vi "MeasureLeakage.vi"(5 "Junction Name":string, 6 "UiDefinition":T1, 7 ".NET Refnum":refnum<k24>, 8 "new file path (Not A Path if cancelled)":path, 9 "appended path":path, 11 ".NET Refnum in":refnum<k24>) -> (0 "error out":errorcluster)   [LabVIEW 2020]
uses:
  UIReferences.ctl
  D:/LabviewDXFViewer/LabviewDXFViewer/bin/Release/LabviewDXFViewer.exe
  LabviewDXFViewer/bin/Release/LabviewDXFViewer.exe
  <vilib>/Utility/file.llb/Write Delimited Spreadsheet (DBL).vi
  <vilib>/Utility/file.llb/Write Delimited Spreadsheet (string).vi
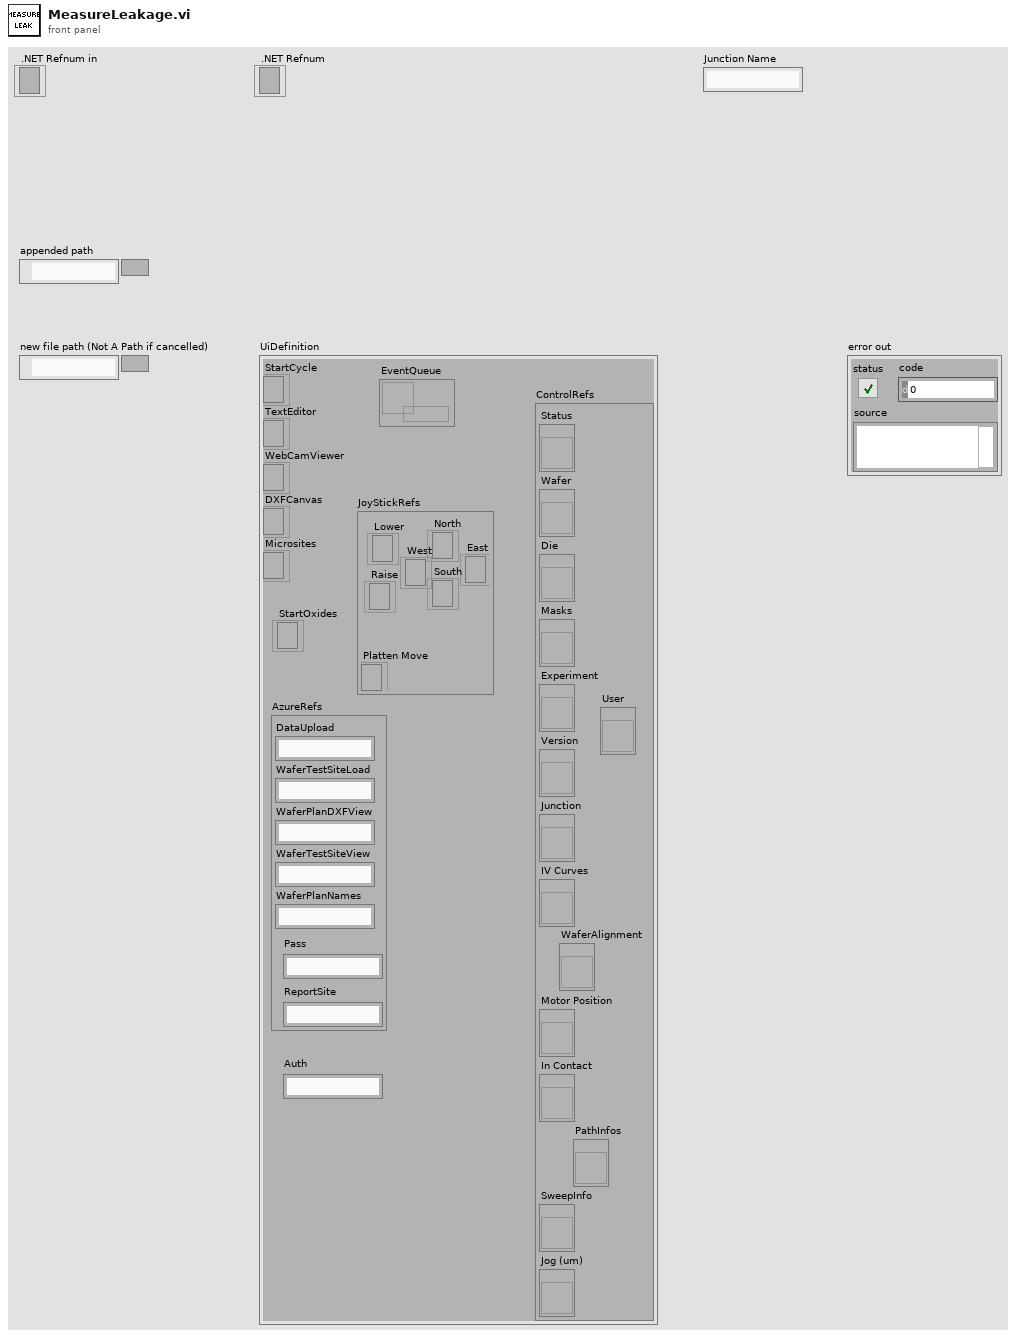
[diagram p1: front panel]
types:
  T1 = typedef "UIReferences.ctl" = cluster{"StartCycle":refnum<k24>, "TextEditor":refnum<k24>, "WebCamViewer":refnum<k24>, "DXFCanvas":refnum<k24>, "Microsites":refnum<k24>, "JoyStickRefs":cluster{"North":refnum<k24>, "Lower":refnum<k24>, "Raise":refnum<k24>, "Platten Move":refnum<k24>, "West":refnum<k24>, "East":refnum<k24>, "South":refnum<k24>}, "AzureRefs":cluster{"DataUpload":string, "WaferTestSiteLoad":string, "WaferPlanDXFView":string, "WaferTestSiteView":string, "WaferPlanNames":string, "Pass":string, "ReportSite":string}, "ControlRefs":cluster{"Status":refnum<vi>, "Wafer":refnum<vi>, "Die":refnum<vi>, "Masks":refnum<vi>, "Experiment":refnum<vi>, "Version":refnum<vi>, "Junction":refnum<vi>, "IV Curves":refnum<vi>, "Motor Position":refnum<vi>, "In Contact":refnum<vi>, "SweepInfo":refnum<vi>, "Jog (um)":refnum<vi>, "PathInfos":refnum<vi>, "User":refnum<vi>, "WaferAlignment":refnum<vi>}, "EventQueue":refnum<queue>, "StartOxides":refnum<k24>, "Auth":string}
  T2 = typedef "CapacitanceInfos.ctl" = cluster{"Conductance":dbl, "CapacitanceIV":dbl, "Intercept":dbl, "CapacitanceSW":dbl, "Sum":dbl, "CapacitanceInfos":T3[], "CapacitancePhase":dbl, "dC/dV":dbl, "Function":string, "OtherInfo":dbl[][]}
  T3 = typedef "CapacitanceRecord.ctl" = cluster{"Freq":dbl, "Vpp":dbl, "PhaseS":dbl, "Irms":dbl, "PhaseC":dbl, "Theta":dbl, "VDrive":dbl, "Capacitance":dbl, "Other":dbl}
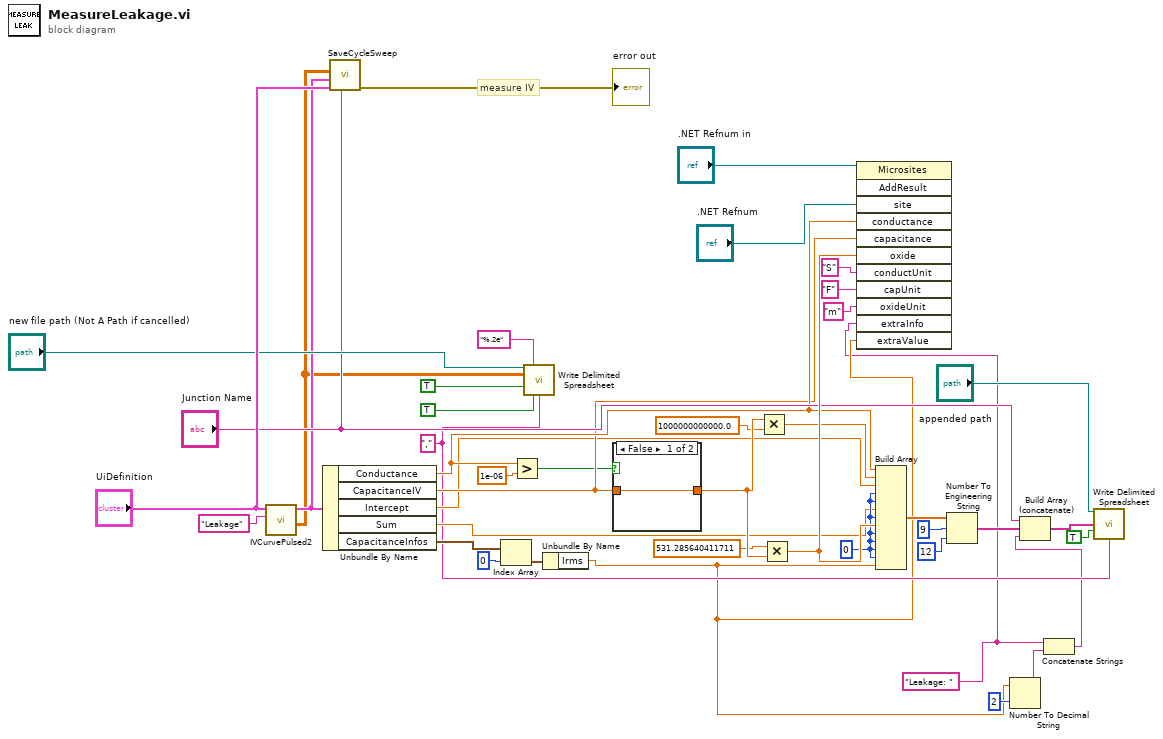
[diagram p0: block diagram]
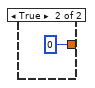
[diagram p2: hidden frame]
diagram:
  w1 = "Leakage: "
  w7 = "," ("delimiter (\\t)")
  w40 = 0
  # "measure IV"
  n1 = call "IVCurvePulsed2.vi"("Program"="Leakage", "UiDefinition"="UiDefinition") -> ("appended array"=w15:dbl[][], "InfoCluster"=w28:T2)  [unwired: 8 in]
  n2 = Unbundle By Name(w28) -> ("Conductance"=w30:dbl, "CapacitanceIV"=w29:dbl, "Intercept"=w18:dbl, "Sum"=w19:dbl, "CapacitanceInfos"=w31:T3[])
  n3 = call "SaveCycleSweep.vi"("JunctionName"="Junction Name", "UiDefinition 2"="UiDefinition", "InfoCluster"=w28, "appended array"=w15) -> ("error out"=→"error out":errorcluster)  [unwired: 7 in]
  n4 = Index Array(array=w31, index=0) -> (element=w33:T3)
  n5 = Greater?(x=w30, y=1e-06) -> (0:w22:bool)
  n6 = call-poly <vilib>:"Write Delimited Spreadsheet.vi"("file path (dialog if empty)"="new file path (Not A Path if cancelled)", "format (%.3f)"="%.2e", "2D data"=w15, "append to file? (new file:F)"=TRUE, "transpose? (no:F)"=TRUE, "delimiter (\\t)"=w7) -> ()  [unwired: 8 in, 2 out]
  n7 = Unbundle By Name(w33) -> ("Irms"=w2:dbl)
  n8 = case shown="False" w22 {
    tunnel: [w44 0] -> w42
    tunnel: w29 -> [w44 _]
    frame False {
    }
    frame True {
    }
  }
  n9 = Multiply(x=w42, y=1000000000000.0) -> (x*y=w20:dbl)
  n10 = Multiply(x=531.285640411711, y=w42) -> (x*y=w43:dbl)
  n11 = invoke class="Microsites" method="AddResult"(reference=".NET Refnum in", "site"=".NET Refnum", "conductance"=w30, "capacitance"=w29, "oxide"=w43, "conductUnit"="S", "capUnit"="F", "oxideUnit"="m" ("interceptUnit"), "extraInfo"=w1, "extraValue"=w2) -> ()  [unwired: 2 in, 12 out]
  n12 = Build Array(w30, w20, w18, w40, w40, w19, w40, w43, w40, w40, w40, w40, w2) -> (w17:dbl[])
  n13 = Number To Engineering String(2:i16 12 ("precision (6)"), 3:i16 9 ("width (-)"), 4:w17) -> (0:w9:string[])  [unwired: 1 in]
  n14 = Number To Decimal String(number=w2, width (-)=i16 2) -> (decimal integer string=w5:string)
  n15 = Concatenate Strings(w1, w5) -> (w3:string)
  n16 = Build Array (concatenate)("Junction Name", w9, w3) -> (w11:string[])
  n17 = call-poly <vilib>:"Write Delimited Spreadsheet.vi"("file path (dialog if empty)"="appended path", "1D data"=w11, "append to file? (new file:F)"=TRUE, "delimiter (\\t)"=w7) -> ()  [unwired: 10 in, 2 out]
